vi "acquire multi waves by LAN.vi"() -> ()   [LabVIEW 2013]
panel:
  in  "address":string="192.168.1.72"
  out "CH1 VOLTS/DIV":string
  out "CH2 VOLTS/DIV":string
  in  "stop":bool
  out "SEC/DIV":string
  out "CH1":string
  out "CH2":string
  out "CH2 SCALE":string
  out "CH2 PROBE":string
  out "Waveform Graph":i32[][](graph)
  out "CH1 PROBE":string
  out "CH1 SCALE":string
  # "1.Fill in the IP Address of your device"
  # "2.Please open the two channels"
  # "3.Please use the stop button to stop the vi"
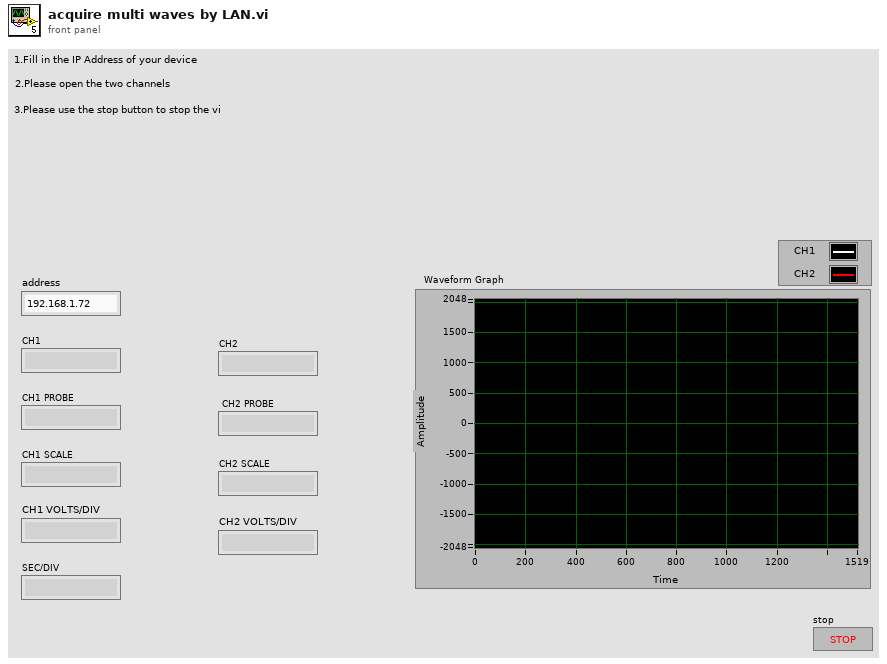
[diagram p1: front panel]
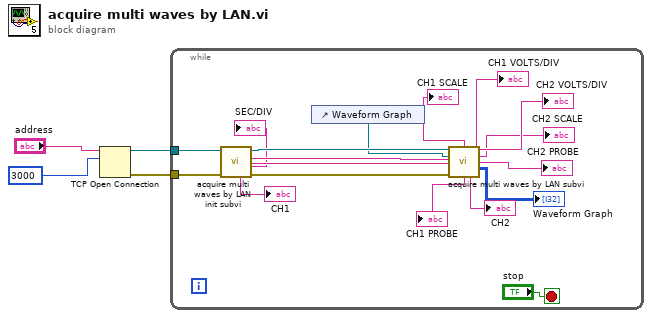
[diagram p0: block diagram]
diagram:
  n1 = TCP Open Connection(address="address", remote port or service name=u16 3000) -> (connection ID=w2:refnum<k5>, error out=w1:errorcluster)  [unwired: 3 in]
  n2 = while {
    tunnel: w2 -> [w20]
    tunnel: w1 -> [w19]
    stop <- "stop" stop-if-true
    n3 = call "acquire multi waves by LAN init subvi.vi"("error in (no error)"=w19, "TCP Network Connection in"=w20) -> ("error out"=w17:errorcluster, "SEC/DIV"=→"SEC/DIV":string, "data out 2"=w21:string, "TCP Network Connection out"=w18:refnum<k5>, "CH1"=→"CH1":string, "data out"=w16:string)  [unwired: 4 in]
    n4 = control-ref of="Waveform Graph"() -> (w13:refnum<vi>)
    n5 = call "acquire multi waves by LAN subvi.vi"("TCP Network Connection in"=w18, "WFGraph Refnum"=w13, 7:"data in"=w16, 9:"data in"=w21, "error in (no error)"=w17) -> ("CH1 SCALE"=→"CH1 SCALE":string, "CH1 VOLTS/DIV"=→"CH1 VOLTS/DIV":string, "CH2 VOLTS/DIV"=→"CH2 VOLTS/DIV":string, "CH2 SCALE"=→"CH2 SCALE":string, "CH2 PROBE"=→"CH2 PROBE":string, "Waveform Graph"=→"Waveform Graph":i32[][], "CH1 PROBE"=→"CH1 PROBE":string, "CH2"=→"CH2":string)  [unwired: 3 in]
  }
